vi "sweep.vi"(6 "Cycles per freq":dbl, 7 "Enable":bool, 9 "Step":dbl, 10 "End frequency":dbl, 11 "Start freqeuncy":dbl) -> ()   [LabVIEW 2023]
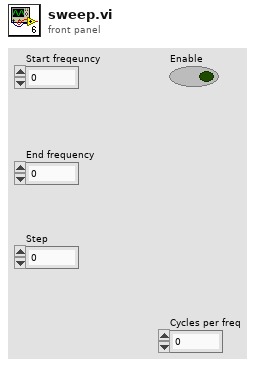
[diagram p1: front panel]
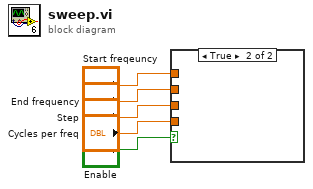
[diagram p0: block diagram]
diagram:
  n1 = case shown="True" "Enable" {
    tunnel: "Start freqeuncy" -> [_ _]
    tunnel: "End frequency" -> [_ _]
    tunnel: "Step" -> [_ _]
    tunnel: "Cycles per freq" -> [_ _]
    frame False {
    }
    frame True {
    }
  }
